vi "ADC Reset Idle Timer.vi"(8 "error in":errorcluster, 10 "set busy (False)":bool, 11 "adc session in":T1={"niScope"={"channel cfg"=[], "sessions"=[], "multi cards"=FALSE, "channels"=0, "type"=enum."n/a", "memory [B/chn]"=0, "ext. clock [Hz]"=0.0, "samples count"=0, "use streaming"=FALSE, "proc setup"={"packet size [smpl]"=0, "current timeout [s]"=0.0, "blk2blk timeout [s]"=0.0, "event time"=timestamp(0 s since 1904-01-01), "temp sampl T [s]"=0.0, "data queue"=refnum, "stop notifier"=refnum, "proc ref"=refnum}, "sample width [B]"=0, "ranges [V]"=[], "trigger setup"={"coupling"=1, "level [V]"=0.0, "slope"=0, "mode"=enum."Immediate"}, "fs [Hz]"=0.0, "bitres [bit]"=0}, "3458A"={"channels"=[], "sync unit"={"VISA"="", "type"=enum."Picotest U6200A"}, "awg unit"={"type"=enum."Agilent 331xxA to 332xxA", "VISA"="", "enable 10MHz ref"=FALSE}, "sync mode"=enum."MASTER-SLAVE, MASTER clocked by TIMER", "streaming mode"=FALSE, "idn mode"=enum."Auto", "sampling mode"=enum."DCV", "Ts [s]"=0.0, "sample memory [B]"=0, "proc setup"={"channel id"=0, "packet size [smpl]"=0, "current timeout [s]"=0.0, "blk2blk timeout [s]"=0.0, "event time"=timestamp(0 s since 1904-01-01), "stop notifier"=refnum, "data queues"=[], "proc refs"=[], "bus semaphore"=refnum}, "sample size [B]"=0, "sample count"=0, "aux data"={"channel id"=0, "valid?"=[], "gain [V]"=[], "timestamp [s]"=[], "Ts [s]"=0.0, "abs timestamp"=timestamp(0 s since 1904-01-01), "t [deg C]"=[]}, "ranges [V]"=[], "aperture [s]"=0.0, "LEVEL trigger"={"edge"=enum."POS", "level [V]"=0.0, "coupling"=enum."DC"}, "trigger mode"=enum."AUTO", "measure temp.?"=FALSE, "disp mesages"=[], "shared bus?"=FALSE, "disable display?"=FALSE, "aper mode"=enum."Manual", "aper rules"=[]}, "dsdll"={"dsdll"={"dsdll path"=path "", "dsdll handle"=[], "output devices"=[], "capture devices"=[]}, "channels"=0, "device id"=0, "channel idns"=[], "proc setup"={"packet size [smpl]"=0, "current timeout [s]"=0.0, "blk2blk timeout [s]"=0.0, "event time"=timestamp(0 s since 1904-01-01), "data queue"=refnum, "stop notifier"=refnum, "proc ref"=refnum}, "samples count"=0, "fs [Hz]"=0.0}, "type"=enum."niScope", "channel idn str"=[], "aux instr idn str"=[], "modified?"=FALSE, "simadc"={"channels"=[], "range [V]"=0.0, "Ts step [s]"=0.0, "time [s]"=0.0, "fs [Hz]"=0.0, "count"=0, "smpl offset"=0, "set count"=0, "bit res"=0}, "force rst?"=FALSE, "exit mode"=enum."Immediate reset", "exit dly"=0.0, "exit tmr"=timestamp(0 s since 1904-01-01), "busy?"=FALSE, "accessed?"=FALSE, "QuADC session"={"channel cfg"=[], "sessions"=[], "multi cards"=FALSE, "channels"=0, "type"=enum."n/a", "memory [B/chn]"=0, "ext. clock [Hz]"=0.0, "samples count"=0, "use streaming"=FALSE, "proc setup"={"packet size [smpl]"=0, "current timeout [s]"=0.0, "blk2blk timeout [s]"=0.0, "event time"=timestamp(0 s since 1904-01-01), "temp sampl T [s]"=0.0, "data queue"=refnum, "stop notifier"=refnum, "proc ref"=refnum}, "sample width [B]"=0, "ranges [V]"=[], "trigger setup"={"coupling"=1, "level [V]"=0.0, "slope"=0, "mode"=enum."Immediate"}, "fs [Hz]"=0.0, "bitres [bit]"=0}} {"QuADC session"."trigger setup"."level [V]" format="%.2f"; "QuADC session"."trigger setup"."coupling" items=["AC"=0, "DC"=1, "HF Reject"=3, "LF Reject"=4, "AC Plus HF Reject"=1001]; "QuADC session"."channel cfg"."Clock fr. (Hz)" min=0.0 format="%#_9p"; "QuADC session"."channel cfg"."Number of JJ" min=1; "QuADC session"."channel cfg"."Range [Vpk]" min=0.0; "QuADC session"."channel cfg"."Channel" min=0; "3458A"."channels"."Range [Vpk]" min=0.0; "niScope"."trigger setup"."level [V]" format="%.2f"; "niScope"."trigger setup"."coupling" items=["AC"=0, "DC"=1, "HF Reject"=3, "LF Reject"=4, "AC Plus HF Reject"=1001]; "niScope"."channel cfg"."Range [Vpk]" min=0.0; "niScope"."channel cfg"."Channel" min=0}) -> (0 "error out":errorcluster, 3 "adc session out":T1={"niScope"={"channel cfg"=[], "sessions"=[], "multi cards"=FALSE, "channels"=0, "type"=enum."n/a", "memory [B/chn]"=0, "ext. clock [Hz]"=0.0, "samples count"=0, "use streaming"=FALSE, "proc setup"={"packet size [smpl]"=0, "current timeout [s]"=0.0, "blk2blk timeout [s]"=0.0, "event time"=timestamp(0 s since 1904-01-01), "temp sampl T [s]"=0.0, "data queue"=refnum, "stop notifier"=refnum, "proc ref"=refnum}, "sample width [B]"=0, "ranges [V]"=[], "trigger setup"={"coupling"=1, "level [V]"=0.0, "slope"=0, "mode"=enum."Immediate"}, "fs [Hz]"=0.0, "bitres [bit]"=0}, "3458A"={"channels"=[], "sync unit"={"VISA"="", "type"=enum."Picotest U6200A"}, "awg unit"={"type"=enum."Agilent 331xxA to 332xxA", "VISA"="", "enable 10MHz ref"=FALSE}, "sync mode"=enum."MASTER-SLAVE, MASTER clocked by TIMER", "streaming mode"=FALSE, "idn mode"=enum."Auto", "sampling mode"=enum."DCV", "Ts [s]"=0.0, "sample memory [B]"=0, "proc setup"={"channel id"=0, "packet size [smpl]"=0, "current timeout [s]"=0.0, "blk2blk timeout [s]"=0.0, "event time"=timestamp(0 s since 1904-01-01), "stop notifier"=refnum, "data queues"=[], "proc refs"=[], "bus semaphore"=refnum}, "sample size [B]"=0, "sample count"=0, "aux data"={"channel id"=0, "valid?"=[], "gain [V]"=[], "timestamp [s]"=[], "Ts [s]"=0.0, "abs timestamp"=timestamp(0 s since 1904-01-01), "t [deg C]"=[]}, "ranges [V]"=[], "aperture [s]"=0.0, "LEVEL trigger"={"edge"=enum."POS", "level [V]"=0.0, "coupling"=enum."DC"}, "trigger mode"=enum."AUTO", "measure temp.?"=FALSE, "disp mesages"=[], "shared bus?"=FALSE, "disable display?"=FALSE, "aper mode"=enum."Manual", "aper rules"=[]}, "dsdll"={"dsdll"={"dsdll path"=path "", "dsdll handle"=[], "output devices"=[], "capture devices"=[]}, "channels"=0, "device id"=0, "channel idns"=[], "proc setup"={"packet size [smpl]"=0, "current timeout [s]"=0.0, "blk2blk timeout [s]"=0.0, "event time"=timestamp(0 s since 1904-01-01), "data queue"=refnum, "stop notifier"=refnum, "proc ref"=refnum}, "samples count"=0, "fs [Hz]"=0.0}, "type"=enum."niScope", "channel idn str"=[], "aux instr idn str"=[], "modified?"=FALSE, "simadc"={"channels"=[], "range [V]"=0.0, "Ts step [s]"=0.0, "time [s]"=0.0, "fs [Hz]"=0.0, "count"=0, "smpl offset"=0, "set count"=0, "bit res"=0}, "force rst?"=FALSE, "exit mode"=enum."Immediate reset", "exit dly"=0.0, "exit tmr"=timestamp(0 s since 1904-01-01), "busy?"=FALSE, "accessed?"=FALSE, "QuADC session"={"channel cfg"=[], "sessions"=[], "multi cards"=FALSE, "channels"=0, "type"=enum."n/a", "memory [B/chn]"=0, "ext. clock [Hz]"=0.0, "samples count"=0, "use streaming"=FALSE, "proc setup"={"packet size [smpl]"=0, "current timeout [s]"=0.0, "blk2blk timeout [s]"=0.0, "event time"=timestamp(0 s since 1904-01-01), "temp sampl T [s]"=0.0, "data queue"=refnum, "stop notifier"=refnum, "proc ref"=refnum}, "sample width [B]"=0, "ranges [V]"=[], "trigger setup"={"coupling"=1, "level [V]"=0.0, "slope"=0, "mode"=enum."Immediate"}, "fs [Hz]"=0.0, "bitres [bit]"=0}} {"QuADC session"."trigger setup"."level [V]" format="%.2f"; "QuADC session"."trigger setup"."coupling" items=["AC"=0, "DC"=1, "HF Reject"=3, "LF Reject"=4, "AC Plus HF Reject"=1001]; "QuADC session"."channel cfg"."Clock fr. (Hz)" min=0.0 format="%#_9p"; "QuADC session"."channel cfg"."Number of JJ" min=1; "QuADC session"."channel cfg"."Range [Vpk]" min=0.0; "QuADC session"."channel cfg"."Channel" min=0; "3458A"."channels"."Range [Vpk]" min=0.0; "niScope"."trigger setup"."level [V]" format="%.2f"; "niScope"."trigger setup"."coupling" items=["AC"=0, "DC"=1, "HF Reject"=3, "LF Reject"=4, "AC Plus HF Reject"=1001]; "niScope"."channel cfg"."Range [Vpk]" min=0.0; "niScope"."channel cfg"."Channel" min=0})   [LabVIEW 2013]
doc: "Reset timeout for delayed reset of digitizer to default state. Set \"set busy\" flag BEFORE using first function of of the driver that accessed digitizer HW. Clear \"set busy\" flag after last HW accessing function call."
uses:
  ADC Session.ctl
  drivers/niScope/niScope Session.ctl
  drivers/niScope/niScope Virtual Channel Config.ctl
  drivers/niScope/niScope Virtual Channel Mode.ctl
  drivers/niScope/niScope Virtual Channel Input Z.ctl
  drivers/niScope/niScope Virtual Channel Coupling.ctl
  drivers/niScope/niScope Type.ctl
  drivers/niScope/niScope Digitizing Process Options.ctl
  drivers/niScope/niScope Data Packet.ctl
  drivers/niScope/niScope Trigger Setup.ctl
  <instrlib>/niScope/Controls/niScope trigger coupling.ctl
  <instrlib>/niScope/Controls/niScope trigger slope.ctl
  drivers/DMM/3458A Digitizer Session.ctl
  drivers/DMM/3458A Virtual Channel Config.ctl
  drivers/Counter/Counter Session.ctl
  drivers/Counter/Counter Type.ctl
  drivers/AWG/AWG Session.ctl
  drivers/AWG/AWG Type.ctl
  drivers/DMM/3458A Sync Mode.ctl
  drivers/DMM/3458A Idn Mode.ctl
  drivers/DMM/3458A Digitizing Low Levels/Configure/Sampling Mode.ctl
  drivers/DMM/3458A Digitizing Process Options.ctl
  drivers/DMM/3458A Data Packet.ctl
  drivers/DMM/3458A Aux Record Data.ctl
  drivers/DMM/3458A Digitizing Low Levels/Configure/Level Setup.ctl
  drivers/DMM/3458A Digitizing Low Levels/Configure/First Sample Trigger.ctl
  drivers/DMM/3458A Aperture Selection Mode.ctl
  drivers/dsdll/DSDLL Session.ctl
  drivers/dsdll/dsdll.lvlibp/dsdll_instance.ctl
  drivers/dsdll/dsdll.lvlibp/dsdll_device_record.ctl
  drivers/dsdll/DSDLL Process Config.ctl
  drivers/dsdll/DSDLL Data Packet.ctl
  ADC Type.ctl
  drivers/simulated_adc/SimAdc Config.ctl
  drivers/simulated_adc/SimAdc Channel Cfg.ctl
  ADC On Close Action.ctl
  drivers/Quatsch_driver/QuADCDriver/QuADC Session.ctl
  drivers/Quatsch_driver/QuADCDriver/QuADC Virtual Channel Config.ctl
  drivers/Quatsch_driver/QuADCDriver/QuADC Virtual Channel Mode.ctl
  drivers/Quatsch_driver/QuADCDriver/QuADC Virtual Channel Input Z.ctl
  drivers/Quatsch_driver/QuADCDriver/QuADC Virtual Channel Coupling.ctl
  drivers/Quatsch_driver/QuADCDriver/QuADC Type.ctl
  drivers/Quatsch_driver/QuADCDriver/QuADC Digitizing Process Options.ctl
  drivers/Quatsch_driver/QuADCDriver/QuADC Data Packet.ctl
  drivers/Quatsch_driver/QuADCDriver/QuADC Trigger Setup.ctl
  drivers/niScope/niScope Virtual Digitizer.lvlib
  drivers/DMM/3458A Virtual Digitizer.lvlib
  drivers/Counter/Counter.lvlib
  drivers/AWG/AWG.lvlib
  drivers/DMM/3458A Digitizing Low Levels/3458A Digitizing Low Levels.lvlib
  drivers/dsdll/dsdll.lvlibp
  drivers/dsdll/DSDLL Virtual Digitizer.lvlib
  drivers/Quatsch_driver/QuADCDriver/QuADC Virtual Digitizer.lvlib
panel:
  # "IP Address"
  # "."
  # "."
  # "."
  # ":"
  # "IP Address"
  # "."
  # "."
  # "."
  # ":"
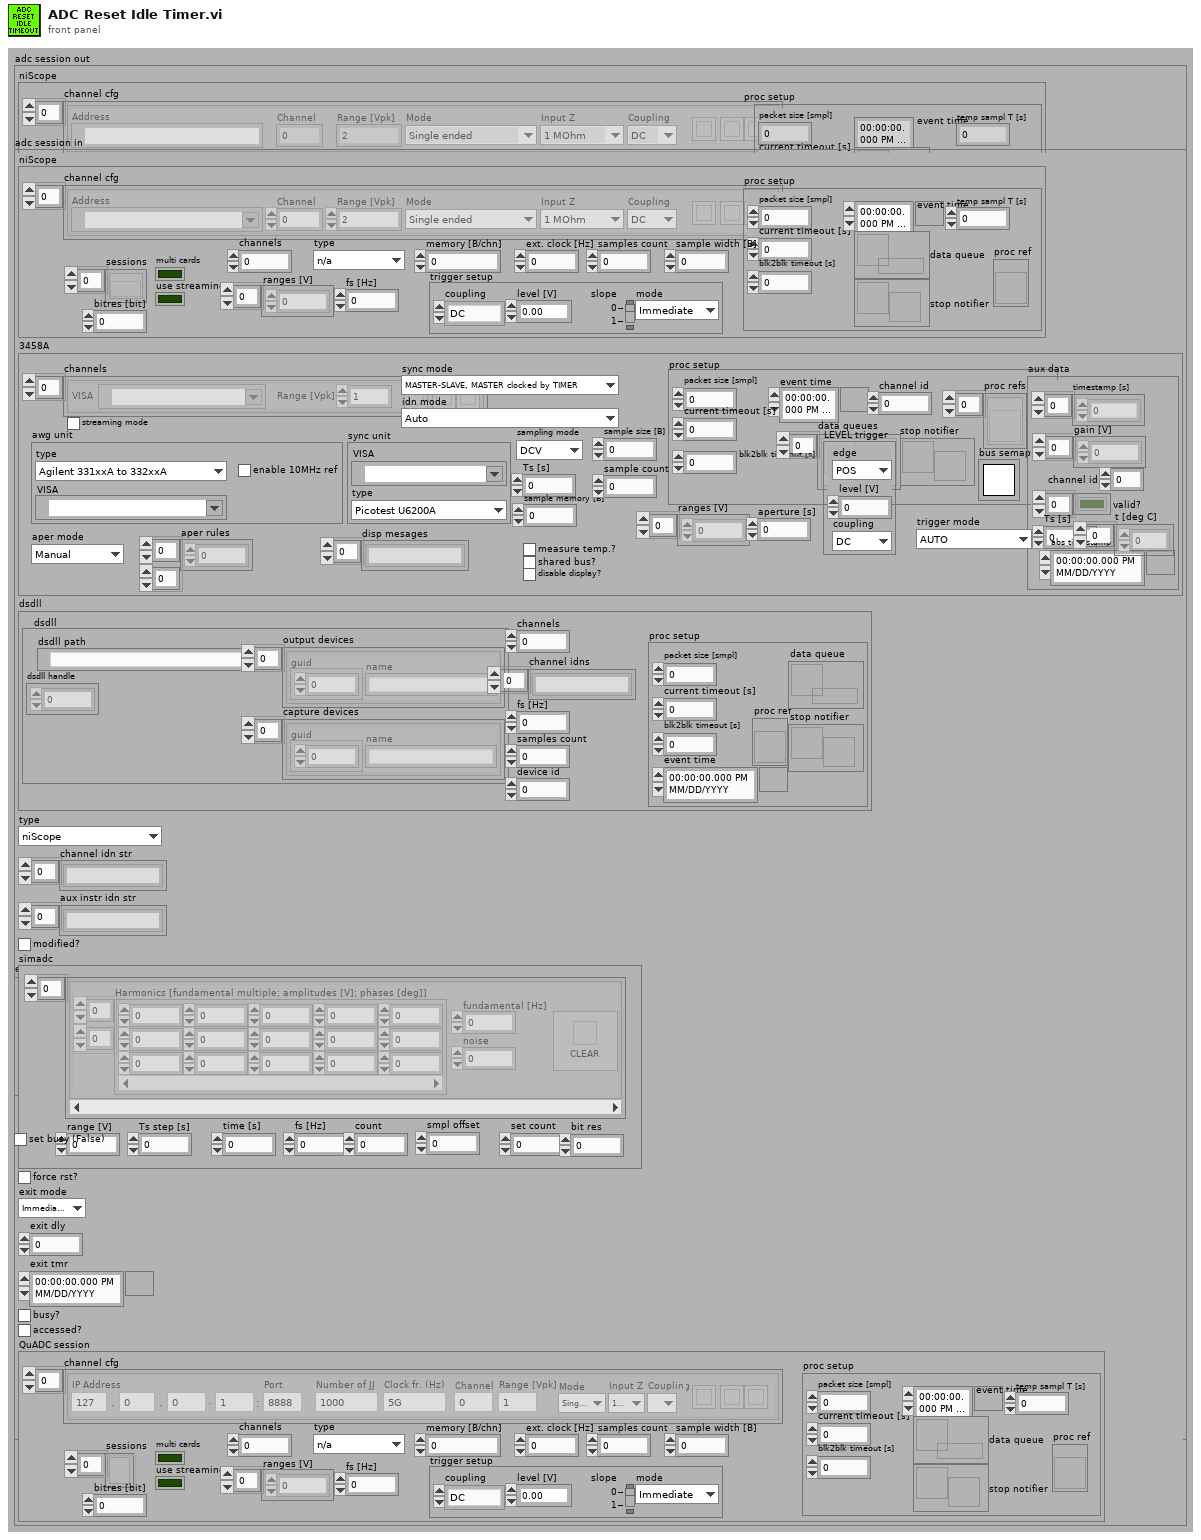
[diagram p1: front panel]
types:
  T1 = typedef "ADC Session.ctl" = cluster{"niScope":T2, "3458A":T12, "dsdll":T27, "type":T31, "channel idn str":string[], "aux instr idn str":string[], "modified?":bool, "simadc":T32, "force rst?":bool, "exit mode":T34, "exit dly":dbl, "exit tmr":timestamp, "busy?":bool, "accessed?":bool, "QuADC session":T35}
  T2 = typedef "niScope Virtual Digitizer.lvlib/niScope Session.ctl" = cluster{"channel cfg":T3[], "sessions":refnum<k20>[], "multi cards":bool, "channels":i32, "type":T7, "memory [B/chn]":i32, "ext. clock [Hz]":dbl, "samples count":i64, "use streaming":bool, "proc setup":T8, "sample width [B]":i32, "ranges [V]":dbl[], "trigger setup":T9, "fs [Hz]":dbl, "bitres [bit]":i32}
  T3 = typedef "niScope Virtual Digitizer.lvlib/niScope Virtual Channel Config.ctl" = cluster{"Address":refnum<k15>, "Channel":i32, "Mode":T4, "Input Z":T5, "Coupling":T6, "Range [Vpk]":dbl, "btn clr":bool, "btn up":bool, "btn down":bool}
  T4 = typedef "niScope Virtual Digitizer.lvlib/niScope Virtual Channel Mode.ctl" = enum16{"Single ended", "Unbal. differential", "Differential"}
  T5 = typedef "niScope Virtual Digitizer.lvlib/niScope Virtual Channel Input Z.ctl" = enum16{"1 MOhm", "50 Ohm"}
  T6 = typedef "niScope Virtual Digitizer.lvlib/niScope Virtual Channel Coupling.ctl" = enum16{"AC", "DC", "GND"}
  T7 = typedef "niScope Virtual Digitizer.lvlib/niScope Type.ctl" = enum16{"n/a", "5922"}
  T8 = typedef "niScope Virtual Digitizer.lvlib/niScope Digitizing Process Options.ctl" = cluster{"packet size [smpl]":i64, "current timeout [s]":dbl, "blk2blk timeout [s]":dbl, "event time":timestamp, "temp sampl T [s]":dbl, "data queue":refnum<queue>, "stop notifier":refnum<notifier>, "proc ref":refnum<vi>}
  T9 = typedef "niScope Virtual Digitizer.lvlib/niScope Trigger Setup.ctl" = cluster{"coupling":T10, "level [V]":dbl, "slope":T11, "mode":enum16{"Immediate", "External", "Level"}}
  T10 = typedef "niScope trigger coupling.ctl" = u16
  T11 = typedef "niScope trigger slope.ctl" = i32
  T12 = typedef "3458A Virtual Digitizer.lvlib/3458A Digitizer Session.ctl" = cluster{"channels":T13[], "sync unit":T14, "awg unit":T16, "sync mode":T18, "streaming mode":bool, "idn mode":T19, "sampling mode":T20, "Ts [s]":dbl, "sample memory [B]":i32, "proc setup":T21, "sample size [B]":i32, "sample count":i32, "aux data":T23, "ranges [V]":dbl[], "aperture [s]":dbl, "LEVEL trigger":T24, "trigger mode":T25, "measure temp.?":bool, "disp mesages":string[], "shared bus?":bool, "disable display?":bool, "aper mode":T26, "aper rules":dbl[][]}
  T13 = typedef "3458A Virtual Digitizer.lvlib/3458A Virtual Channel Config.ctl" = cluster{"VISA":refnum<visa-resource-name>, "Range [Vpk]":dbl, "btn clr":bool, "btn up":bool, "btn down":bool}
  T14 = typedef "Counter.lvlib/Counter Session.ctl" = cluster{"VISA":refnum<visa-resource-name>, "type":T15}
  T15 = typedef "Counter.lvlib/Counter Type.ctl" = enum16{"Picotest U6200A", "dummy"}
  T16 = typedef "AWG.lvlib/AWG Session.ctl" = cluster{"type":T17, "VISA":refnum<visa-resource-name>, "enable 10MHz ref":bool}
  T17 = typedef "AWG.lvlib/AWG Type.ctl" = enum16{"Agilent 331xxA to 332xxA", "Agilent 335xxA to 336xxA", "Tektronix AFG3101C", "dummy"}
  T18 = typedef "3458A Virtual Digitizer.lvlib/3458A Sync Mode.ctl" = enum16{"MASTER-SLAVE, MASTER clocked by TIMER", "MASTER-SLAVE, MASTER clocked by AWG", "ALL clocked by AWG", "MASTER-SLAVE, ALL clocked by TIMER", "ALL clocked by AWG with DFLL"}
  T19 = typedef "3458A Virtual Digitizer.lvlib/3458A Idn Mode.ctl" = enum16{"Auto", "Sequential (chn A, chn B, ...)", "From calibration string"}
  T20 = typedef "3458A Virtual Digitizer.lvlib/3458A Digitizing Low Levels.lvlib/Sampling Mode.ctl" = enum16{"DCV", "DSDC", "DSAC"}
  T21 = typedef "3458A Virtual Digitizer.lvlib/3458A Digitizing Process Options.ctl" = cluster{"channel id":i32, "packet size [smpl]":i32, "current timeout [s]":dbl, "blk2blk timeout [s]":dbl, "event time":timestamp, "stop notifier":refnum<notifier>, "data queues":refnum<queue>[], "proc refs":refnum<vi>[], "bus semaphore":T22}
  T22 = typedef "Semaphore RefNum" = refnum<k1>
  T23 = typedef "3458A Virtual Digitizer.lvlib/3458A Aux Record Data.ctl" = cluster{"channel id":i32, "valid?":bool[], "gain [V]":dbl[], "timestamp [s]":dbl[], "Ts [s]":dbl, "abs timestamp":timestamp, "t [deg C]":dbl[]}
  T24 = typedef "3458A Virtual Digitizer.lvlib/3458A Digitizing Low Levels.lvlib/Level Setup.ctl" = cluster{"edge":enum16{"POS", "NEG"}, "level [V]":dbl, "coupling":enum16{"DC", "AC"}}
  T25 = typedef "3458A Virtual Digitizer.lvlib/3458A Digitizing Low Levels.lvlib/First Sample Trigger.ctl" = enum16{"AUTO", "EXT", "SYN", "SGL", "HOLD", "LEVEL"}
  T26 = typedef "3458A Virtual Digitizer.lvlib/3458A Aperture Selection Mode.ctl" = enum16{"Manual", "Maximum", "Table"}
  T27 = typedef "DSDLL Virtual Digitizer.lvlib/DSDLL Session.ctl" = cluster{"dsdll":T28, "channels":i32, "device id":i32, "channel idns":string[], "proc setup":T30, "samples count":i32, "fs [Hz]":dbl}
  T28 = typedef "dsdll.lvlibp/dsdll_instance.ctl" = cluster{"dsdll path":path, "dsdll handle":u8[], "output devices":T29[], "capture devices":T29[]}
  T29 = typedef "dsdll.lvlibp/dsdll_device_record.ctl" = cluster{"guid":u8[], "name":string}
  T30 = typedef "DSDLL Virtual Digitizer.lvlib/DSDLL Process Config.ctl" = cluster{"packet size [smpl]":i32, "current timeout [s]":dbl, "blk2blk timeout [s]":dbl, "event time":timestamp, "data queue":refnum<queue>, "stop notifier":refnum<notifier>, "proc ref":refnum<vi>}
  T31 = typedef "ADC Type.ctl" = enum16{"niScope", "3458A", "DirectSound DLL", "dummy", "QuADC"}
  T32 = typedef "SimAdc Config.ctl" = cluster{"channels":T33[], "range [V]":dbl, "Ts step [s]":dbl, "time [s]":dbl, "fs [Hz]":dbl, "count":i64, "smpl offset":i64, "set count":i64, "bit res":i32}
  T33 = typedef "SimAdc Channel Cfg.ctl" = cluster{"harmonics":dbl[][], "btn clear":bool, "noise":dbl, "fundamental [Hz]":dbl}
  T34 = typedef "ADC On Close Action.ctl" = enum16{"Immediate reset", "Delayed reset"}
  T35 = typedef "QuADC Virtual Digitizer.lvlib/QuADC Session.ctl" = cluster{"channel cfg":T36[], "sessions":refnum<k5>[], "multi cards":bool, "channels":i32, "type":T40, "memory [B/chn]":i32, "ext. clock [Hz]":dbl, "samples count":i64, "use streaming":bool, "proc setup":T41, "sample width [B]":i32, "ranges [V]":dbl[], "trigger setup":T42, "fs [Hz]":dbl, "bitres [bit]":i32}
  T36 = typedef "QuADC Virtual Digitizer.lvlib/QuADC Virtual Channel Config.ctl" = cluster{"Channel":i32, "Mode":T37, "Input Z":T38, "Coupling":T39, "Range [Vpk]":dbl, "btn clr":bool, "btn up":bool, "btn down":bool, "IP address A":u8, "IP address B":u8, "IP address C":u8, "IP address D":u8, "Port":u16, "Number of JJ":u32, "Clock fr. (Hz)":dbl}
  T37 = typedef "QuADC Virtual Digitizer.lvlib/QuADC Virtual Channel Mode.ctl" = enum16{"Single ended", "Unbal. differential", "Differential"}
  T38 = typedef "QuADC Virtual Digitizer.lvlib/QuADC Virtual Channel Input Z.ctl" = enum16{"1 MOhm", "50 Ohm"}
  T39 = typedef "QuADC Virtual Digitizer.lvlib/QuADC Virtual Channel Coupling.ctl" = enum16{"AC", "DC", "GND"}
  T40 = typedef "QuADC Virtual Digitizer.lvlib/QuADC Type.ctl" = enum16{"n/a", "v1"}
  T41 = typedef "QuADC Virtual Digitizer.lvlib/QuADC Digitizing Process Options.ctl" = cluster{"packet size [smpl]":i64, "current timeout [s]":dbl, "blk2blk timeout [s]":dbl, "event time":timestamp, "temp sampl T [s]":dbl, "data queue":refnum<queue>, "stop notifier":refnum<notifier>, "proc ref":refnum<vi>}
  T42 = typedef "QuADC Virtual Digitizer.lvlib/QuADC Trigger Setup.ctl" = cluster{"coupling":T10, "level [V]":dbl, "slope":T11, "mode":enum16{"Immediate", "External", "Level"}}
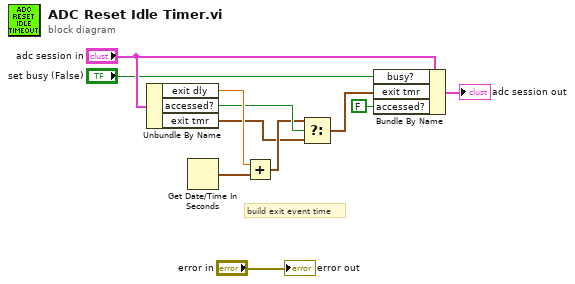
[diagram p0: block diagram]
diagram:
  # "build exit event time"
  n1 = Unbundle By Name("adc session in") -> ("exit dly"=w9:dbl, "accessed?"=w5:bool, "exit tmr"=w3:timestamp)
  n2 = Get Date/Time In Seconds() -> (seconds since 1Jan1904=w8:timestamp)
  n3 = Add(x=w9, y=w8) -> (x+y=w4:timestamp)
  n4 = Select(t=w4, s=w5, f=w3) -> (s? t:f=w2:timestamp)
  n5 = Bundle By Name(cluster="adc session in", "busy?"="set busy (False)", "exit tmr"=w2, "accessed?"=FALSE) -> (→"adc session out":T1)
  "error out" <- "error in"
